vi "Remove Not Tested Data.vi"(11 "Table":T1[](array[typedef])) -> (3 "Table 2":T1[](array[typedef]))   [LabVIEW 2011]
uses:
  CGI SimpleStat Results.ctl
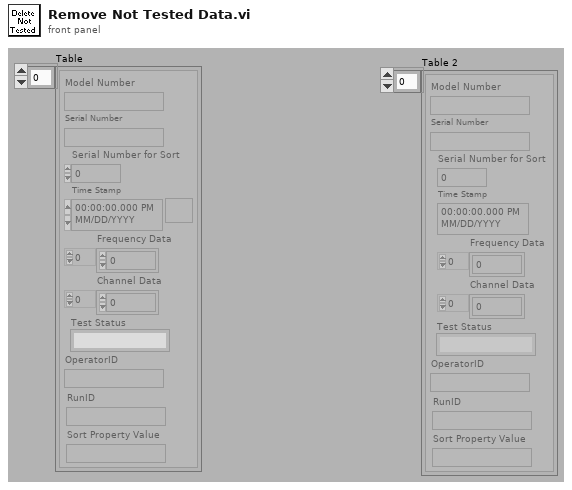
[diagram p1: front panel]
types:
  T1 = typedef "CGI SimpleStat Results.ctl" = cluster{"Model Number":string, "Serial Number for Sort":i32, "Serial Number":string, "Time Stamp":timestamp, "Channel Data":dbl[], "Test Status":string, "OperatorID":string, "Frequency Data":dbl[], "RunID":string, "Sort Property Value":string}
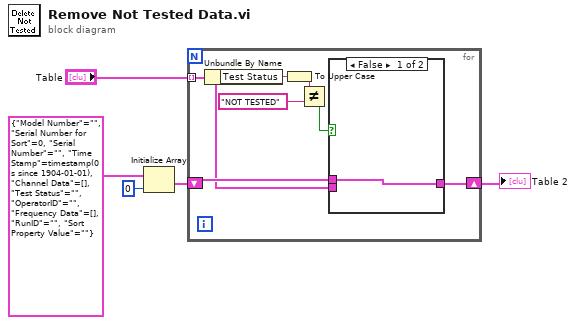
[diagram p0: block diagram]
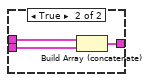
[diagram p2: hidden frame]
diagram:
  n1 = Initialize Array(T1 {"Model Number"="", "Serial Number for Sort"=0, "Serial Number"="", "Time Stamp"=timestamp(0 s since 1904-01-01), "Channel Data"=[], "Test Status"="", "OperatorID"="", "Frequency Data"=[], "RunID"="", "Sort Property Value"=""} ("Sample Results"), 0 ("dimension size")) -> (w3:T1[])
  n2 = for {
    tunnel: "Table" -> [w8] mode=indexing
    shift-right: [w10] -> w1
    shift-left: w3 -> [w9]
    n3 = Unbundle By Name(w8) -> ("Test Status"=w11:string)
    n4 = To Upper Case(1:w11) -> (0:w6:string)
    n5 = Not Equal?(x=w6, y="NOT TESTED") -> (x != y?=w7:bool)
    n6 = case shown="False" w7 {
      tunnel: [w13 w16] -> w10
      tunnel: w9 -> [w13 w15]
      tunnel: w8 -> [_ w14]
      frame False {
      }
      frame True {
        n7 = Build Array (concatenate)(w15, w14) -> (w16:T1[])
      }
    }
  }
  "Table 2" <- w1
